vi "CMC_Homework06_Main.vi"() -> ()   [LabVIEW 2013]
uses:
  <vilib>/Utility/error.llb/DialogType.ctl
  <vilib>/Utility/error.llb/Error Cluster From Error Code.vi
  <vilib>/ErrorRing/Error Ring.xnode
panel:
  out "Final Letter Grade":string
  in  "Use Grad Distrib":bool
  in  "Grades, Contribution Percent":string[][](table)
  in  "Grade Cutoffs":T1={"Letter Grade D Cutoff"=60.0, "Letter Grade C Cutoff"=70.0, "Letter Grade B Cutoff"=80.0, "Letter Grade A Cutoff"=90.0}
  # "Assignment"
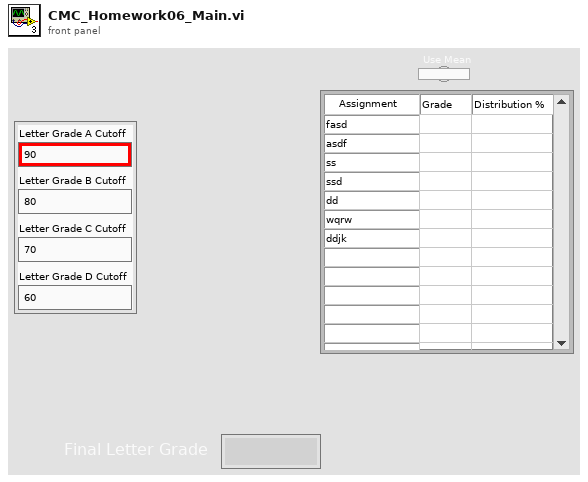
[diagram p1: front panel]
types:
  T1 = cluster{"Letter Grade D Cutoff":dbl, "Letter Grade C Cutoff":dbl, "Letter Grade B Cutoff":dbl, "Letter Grade A Cutoff":dbl}
  T2 = typedef "DialogType.ctl" = u16
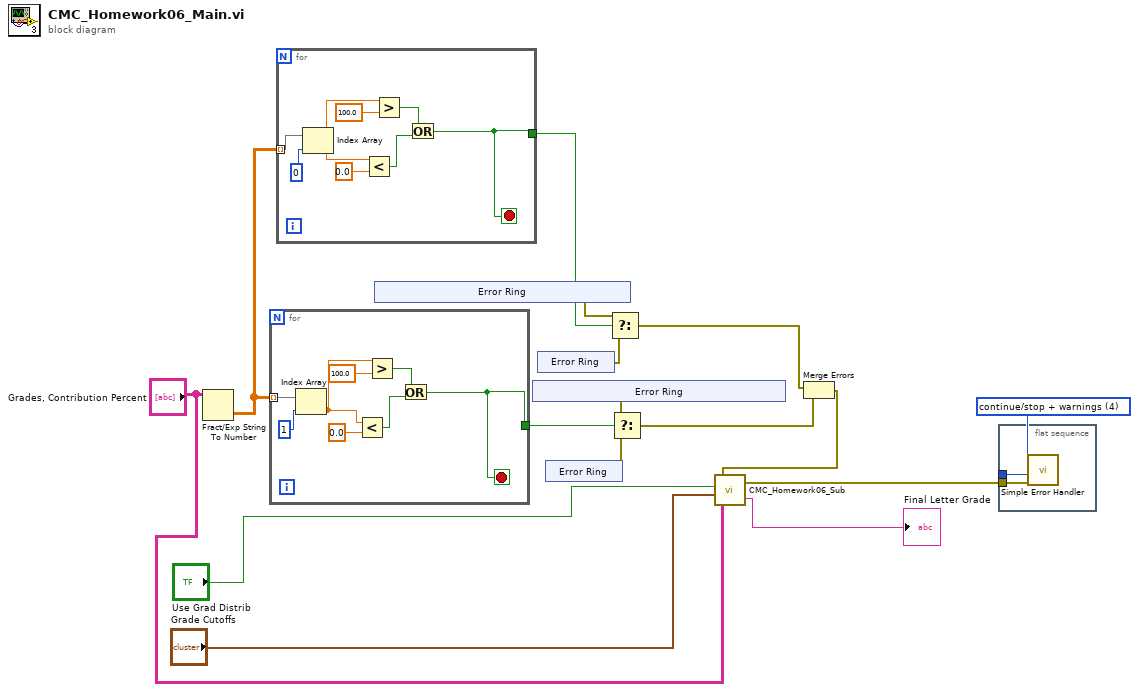
[diagram p0: block diagram]
diagram:
  w1 = T2 4 items=["no dialog", "OK message", "continue or stop message", "OK message + warnings", "continue/stop + warnings"] ("type of dialog (OK msg:1)")
  n1 = Fract/Exp String To Number(string="Grades, Contribution Percent") -> (number=w11:dbl[][])  [unwired: 3 in, 1 out]
  n2 = for {
    tunnel: [w20] -> w9
    tunnel: w11 -> [w18] mode=indexing
    stop <- w20 stop-if-true
    n3 = Index Array(array=w18, index=1) -> (element=w17:dbl)
    n4 = Less?(x=w17, y=0.0) -> (x < y?=w21:bool)
    n5 = Greater?(x=w17, y=100.0) -> (0:w22:bool)
    n6 = Or(x=w22, y=w21) -> (x .or. y?=w20:bool)
  }
  n7 = for {
    tunnel: w11 -> [w30] mode=indexing
    tunnel: [w26] -> w16
    stop <- w26 stop-if-true
    n8 = Index Array(array=w30, index=0) -> (element=w29:dbl)
    n9 = Less?(x=w29, y=0.0) -> (x < y?=w27:bool)
    n10 = Greater?(x=w29, y=100.0) -> (0:w28:bool)
    n11 = Or(x=w28, y=w27) -> (x .or. y?=w26:bool)
  }
  n12 = xnode "Error Ring"() -> ("error out"=w15:errorcluster)
  n13 = xnode "Error Ring"() -> ("error out"=w6:errorcluster)
  n14 = xnode "Error Ring"() -> ("error out"=w10:errorcluster)
  n15 = xnode "Error Ring"() -> ("error out"=w8:errorcluster)
  n16 = Select(t=w15, s=w16, f=w10) -> (s? t:f=w7:errorcluster)
  n17 = Select(t=w6, s=w9, f=w8) -> (s? t:f=w5:errorcluster)
  n18 = Merge Errors(w7, w5) -> (w4:errorcluster)
  n19 = call "CMC_Homework06_Sub.vi"("Grades"="Grades, Contribution Percent", "Grade Cutoffs"="Grade Cutoffs", "Use Grade Distrib"="Use Grad Distrib", "error in (no error)"=w4) -> ("String"=→"Final Letter Grade":string, "error out"=w2:errorcluster)
  n20 = flat-sequence {
    tunnel: w2 -> [w34]
    tunnel: w1 -> [w33]
    frame #0 {
      n21 = call <vilib>:"Simple Error Handler.vi"("type of dialog (OK msg:1)"=w33, "error in (no error)"=w34) -> ()  [unwired: 3 in, 5 out]
    }
  }
